vi "Read TopRef.vi"(8 "error in (no error)":errorcluster, 11 "UIActorTop2 in":refnum<class "SCLB_Template.lvclass">) -> (0 "error out":errorcluster, 2 "TopRef":T1, 3 "UIActorTop2 out":refnum<class "SCLB_Template.lvclass">)   [LabVIEW 2021, in "SCLB_Template.lvclass"]
uses:
  SCLB_Template.lvclass
  TopRef.ctl
  SCLB_Template.lvclass/SCLB_Template.ctl
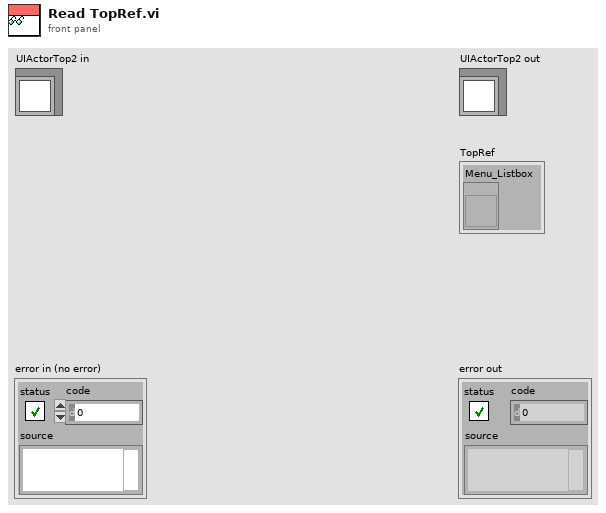
[diagram p1: front panel]
types:
  T1 = typedef "SCLB_Template.lvclass/TopRef.ctl" = cluster{"Menu_Listbox":refnum<vi>}
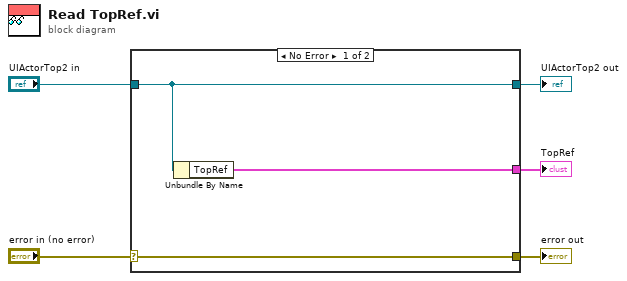
[diagram p0: block diagram]
diagram:
  n1 = case shown="No Error" "error in (no error)" {
    selector: "error in (no error)" -> [w8 w9]
    tunnel: [w8 w9] -> w4
    tunnel: [w7 w10] -> w2
    tunnel: "UIActorTop2 in" -> [w7 w10]
    tunnel: [w6 _] -> w1
    frame No Error {
      n2 = Unbundle By Name(w7) -> ("TopRef"=w6:T1)
    }
    frame Error {
    }
  }
  "error out" <- w4
  "UIActorTop2 out" <- w2
  "TopRef" <- w1
